vi "Get Platform.vi"(11 "IO":T2) -> (3 "IO":T1)   [LabVIEW 2020, in "LMH-LINX.lvlib"]
uses:
  LMH-LINX.lvlib
  Type Defs/User Platform.ctl
  Type Defs/Platform.ctl
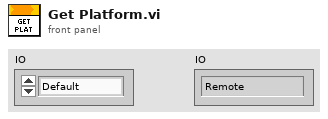
[diagram p1: front panel]
types:
  T1 = typedef "LMH-LINX.lvlib/Platform.ctl" = enum16{"Remote", "Local"}
  T2 = typedef "LMH-LINX.lvlib/User Platform.ctl" = enum16{"Default", "Remote", "Local"}
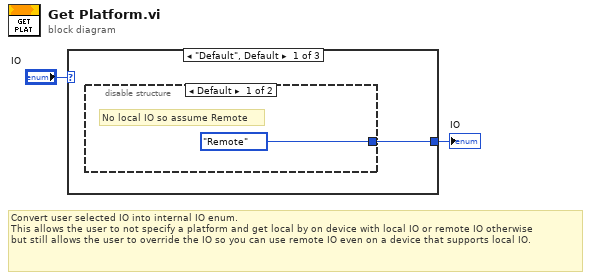
[diagram p0: block diagram]
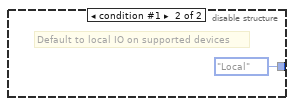
[diagram p2: hidden frame]
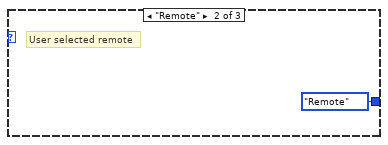
[diagram p3: hidden frame]
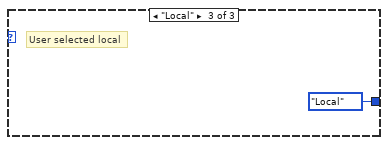
[diagram p4: hidden frame]
diagram:
  # "Convert user selected IO into internal IO enum.\nThis allows the user to not specify a platform and get local by on device with local IO or remote IO otherwise\nbut still allows the user to override the IO so you can use remote IO even on a device that supports local IO."
  n1 = case shown="\"Default\", Default" "IO" {
    tunnel: [w3 Platform."Remote" ("Platform") Platform."Local" ("Platform")] -> w1
    frame "Default", Default {
      n2 = disable-structure shown="Default" {
        disable-tunnel: [Platform."Remote" ("Platform") Platform."Local" ("Platform")] -> w3
        frame condition #0 (active) {
          # "No local IO so assume Remote"
        }
        frame condition #1 {
          # "Default to local IO on supported devices"
        }
      }
    }
    frame "Remote" {
      # "User selected remote"
    }
    frame "Local" {
      # "User selected local"
    }
  }
  "IO" <- w1
